vi "CRYPIC CLOSE FRAME.vi"(10 "tFrame":T2) -> ()   [LabVIEW 2013]
uses:
  <vilib>/Utility/miscctls.llb/LVRectTypeDef.ctl
  CRYMain Sub Window Global.vi
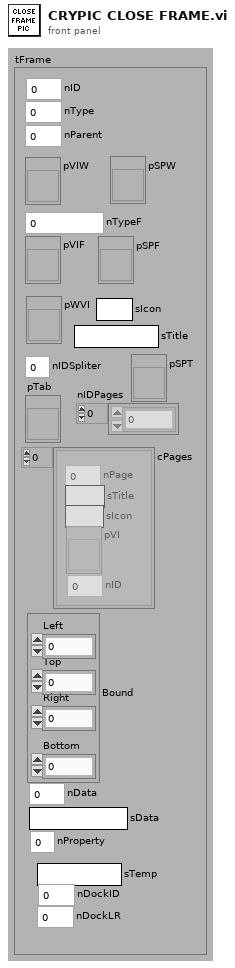
[diagram p1: front panel]
types:
  T1 = typedef "LVRectTypeDef.ctl" = cluster{"Left":i16, "Top":i16, "Right":i16, "Bottom":i16}
  T2 = cluster{"nType":i32, "nParent":i32, "pVIW":refnum<vi>, "pSPW":refnum<vi>, "nTypeF":i32, "pVIF":refnum<vi>, "pSPF":refnum<vi>, "nIDSpliter":i32, "nProperty":i32, "Bound":T1, "nID":i32, "nData":i32, "sData":string, "pWVI":refnum<vi>, "sTitle":string, "cPages":cluster{"nPage":i32, "sTitle":string, "sIcon":string, "pVI":refnum<vi>, "nID":i32}[], "pTab":refnum<vi>, "nIDPages":i32[], "pSPT":refnum<vi>, "sTemp":string, "nDockID":i32, "nDockLR":i32, "sIcon":string}
  T3 = enum32{"Invalid", "Standard", "Closed", "Hidden", "Minimized", "Maximized"}
  T4 = cluster{"nID":i32[], "Frame":cluster{"nType":i32, "nParent":i32, "pVIW":refnum<vi>, "pSPW":refnum<vi>, "nTypeF":i32, "pVIF":refnum<vi>, "pSPF":refnum<vi>, "nIDSpliter":i32, "nProperty":i32, "Bound":T1, "nID":i32, "nData":i32, "sData":string, "pWVI":refnum<vi>, "sTitle":string, "cPages":cluster{"nPage":i32, "sTitle":string, "sIcon":string, "pVI":refnum<vi>, "nID":i32}[], "pTab":refnum<vi>, "nIDPages":i32[], "pSPT":refnum<vi>, "sTemp":string, "nDockID":i32, "nDockLR":i32, "sIcon":string}[]}
  T5 = cluster{"nType":i32, "nParent":i32, "pVIW":refnum<vi>, "pSPW":refnum<vi>, "nTypeF":i32, "pVIF":refnum<vi>, "pSPF":refnum<vi>, "nIDSpliter":i32, "nProperty":i32, "Bound":T1, "nID":i32, "nData":i32, "sData":string, "pWVI":refnum<vi>, "sTitle":string, "cPages":cluster{"nPage":i32, "sTitle":string, "sIcon":string, "pVI":refnum<vi>, "nID":i32}[], "pTab":refnum<vi>, "nIDPages":i32[], "pSPT":refnum<vi>, "sTemp":string, "nDockID":i32, "nDockLR":i32, "sIcon":string}[]
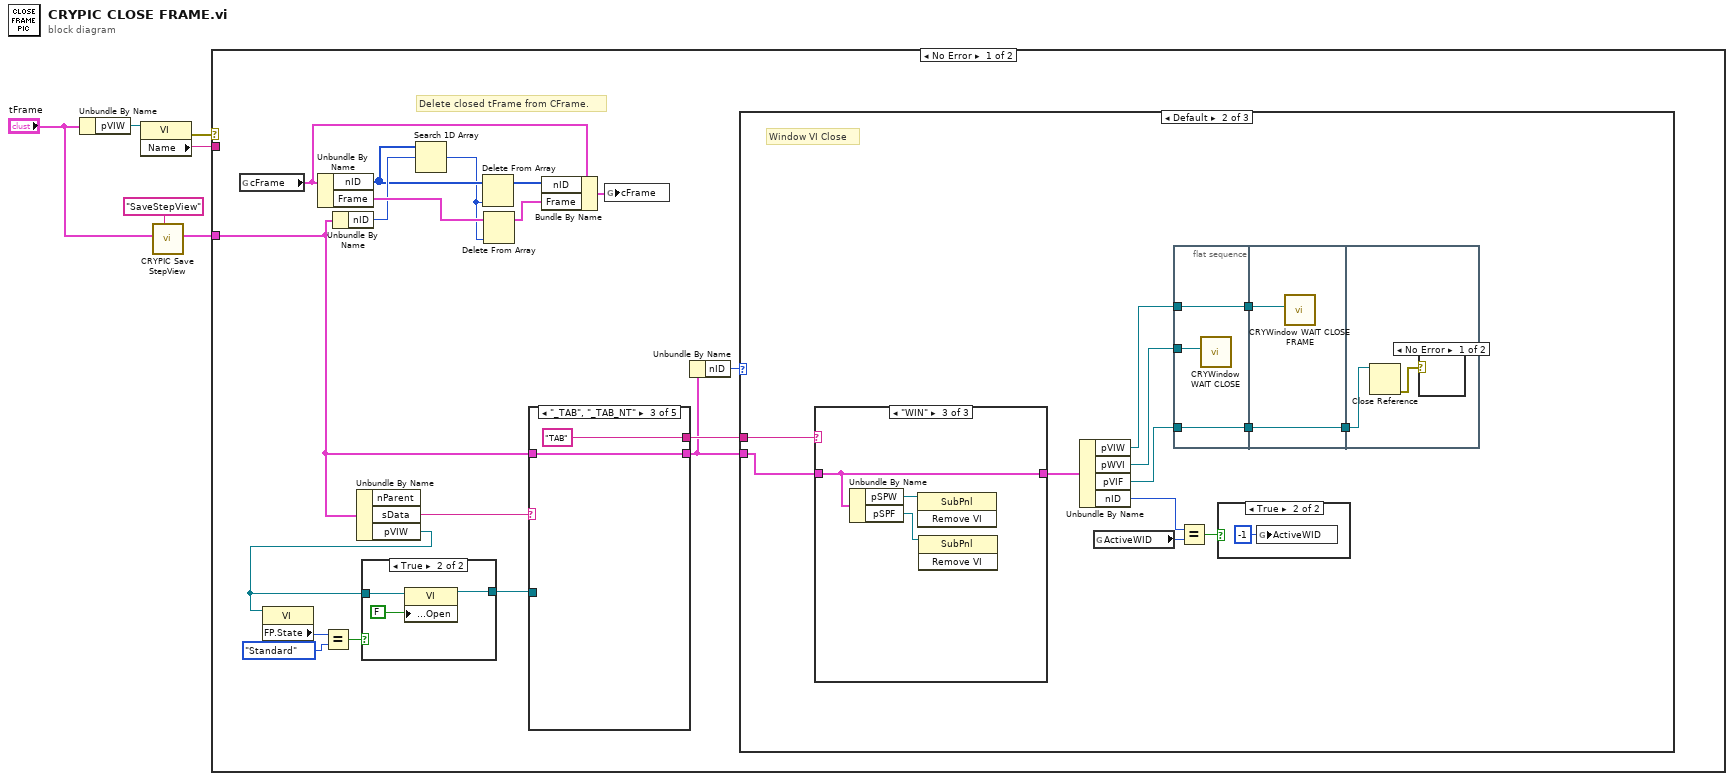
[diagram p0: block diagram]
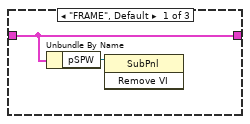
[diagram p4: hidden frame]
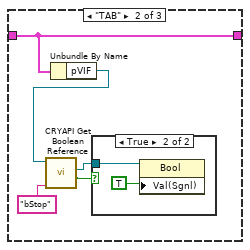
[diagram p5: hidden frame]
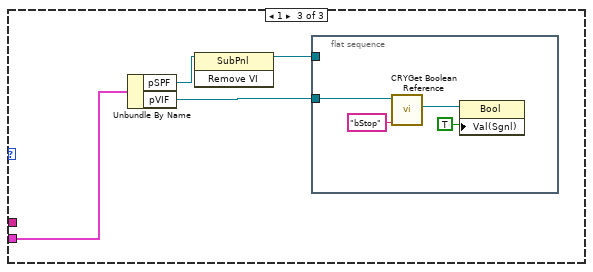
[diagram p8: hidden frame]
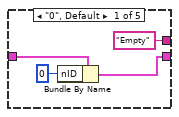
[diagram p10: hidden frame]
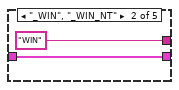
[diagram p11: hidden frame]
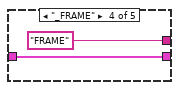
[diagram p12: hidden frame]
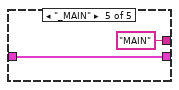
[diagram p13: hidden frame]
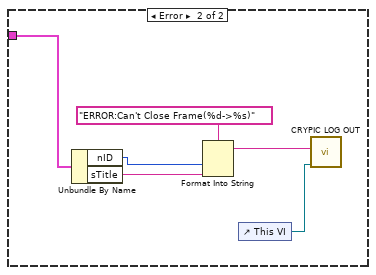
[diagram p14: hidden frame]
diagram:
  n1 = Unbundle By Name("tFrame") -> ("pVIW"=w6:refnum<vi>)
  n2 = property class="VI"(reference=w6) -> (error out=w5:errorcluster, "Name"=w4:string)  [unwired: 1 in, 1 out]
  n3 = call "CRYPIC Save StepView.vi"("sAction"="SaveStepView", "tFrame"="tFrame") -> ("tFrame_Out"=w2:T2)  [unwired: 9 in]
  n4 = case shown="No Error" w5 {
    tunnel: w4 -> [_ _]
    tunnel: w2 -> [w7 w81]
    frame No Error {
      # "Delete closed tFrame from CFrame."
      n5 = global read "CRYMain Sub Window Global.vi" "cFrame"() -> (w23:T4)
      n6 = Unbundle By Name(w23) -> ("nID"=w18:i32[], "Frame"=w24:T5)
      n7 = Unbundle By Name(w7) -> ("nID"=w19:i32)
      n8 = Unbundle By Name(w7) -> ("sData"=w11:string, "pVIW"=w12:refnum<vi>)  [unwired: 1 out]
      n9 = property class="VI"(reference=w12) -> ("FP.State"=w14:T3)  [unwired: 1 in, 2 out]
      n10 = Equal?(x=w14, y=T3."Standard" ("Front Panel Window:State")) -> (x = y?=w13:bool)
      n11 = case shown="True" w13 {
        tunnel: [w65 w67] -> w16
        tunnel: w12 -> [w65 w66]
        frame False {
        }
        frame True {
          n12 = property class="VI"(reference=w66, "Front Panel.Open"=FALSE ("Front Panel Window:Open")) -> (reference out=w67:refnum<vi>)  [unwired: 1 in, 1 out]
        }
      }
      n13 = Search 1D Array(1D array=w18, element=w19) -> (index of element=w17:i32)  [unwired: 1 out]
      n14 = Delete From Array(array=w18, index=w17) -> (array with subset deleted=w22:i32[])  [unwired: 1 in, 1 out]
      n15 = Delete From Array(array=w24, index=w17) -> (array with subset deleted=w21:T5)  [unwired: 1 in, 1 out]
      n16 = case shown="\"_TAB\", \"_TAB_NT\"" w11 {
        tunnel: w7 -> [w72 w74 w75 w77 w79]
        tunnel: [w70 w74 w75 w77 w79] -> w9
        tunnel: w16 -> [_ _ _ _ _]
        tunnel: ["Empty" ("sAction") "WIN" ("sAction") "TAB" ("sAction") "FRAME" ("sAction") "MAIN" ("sAction")] -> w10
        frame "0", Default {
          n17 = Bundle By Name(cluster=w72, "nID"=0) -> (w70:T2)
        }
        frame "_WIN", "_WIN_NT" {
        }
        frame "_TAB", "_TAB_NT" {
        }
        frame "_FRAME" {
        }
        frame "_MAIN" {
        }
      }
      n18 = Bundle By Name(cluster=w23, "nID"=w22, "Frame"=w21) -> (w20:T4)
      n19 = global write "CRYMain Sub Window Global.vi" "cFrame"(w20) -> ()
      n20 = Unbundle By Name(w9) -> ("nID"=w8:i32)
      n21 = case shown="Default" w8 {
        tunnel: w9 -> [_ w25 w60]
        tunnel: w10 -> [_ w33 _]
        frame 0 {
        }
        frame Default {
          # "Window VI Close"
          n22 = case shown="\"WIN\"" w33 {
            tunnel: w25 -> [w45 w50 w55]
            tunnel: [w45 w50 w55] -> w26
            frame "FRAME", Default {
              n23 = Unbundle By Name(w45) -> ("pSPW"=w44:refnum<vi>)
              n24 = invoke class="SubPnl" method="Remove VI"(reference=w44) -> ()  [unwired: 2 in, 3 out]
            }
            frame "TAB" {
              n25 = Unbundle By Name(w50) -> ("pVIF"=w46:refnum<vi>)
              n26 = call "CRYAPI Get Boolean Reference.vi"("Label Name"="bStop", "VI Refnum"=w46) -> ("Boolean"=w47:bool, "Boolean Ref"=w49:refnum<vi>)  [unwired: 8 out]
              n27 = case shown="True" w47 {
                tunnel: w49 -> [_ w52]
                frame False {
                }
                frame True {
                  n28 = property class="Bool"(reference=w52, "Val(Sgnl)"=TRUE) -> ()  [unwired: 1 in, 2 out]
                }
              }
            }
            frame "WIN" {
              n29 = Unbundle By Name(w55) -> ("pSPW"=w54:refnum<vi>, "pSPF"=w53:refnum<vi>)
              n30 = invoke class="SubPnl" method="Remove VI"(reference=w54) -> ()  [unwired: 2 in, 3 out]
              n31 = invoke class="SubPnl" method="Remove VI"(reference=w53) -> ()  [unwired: 2 in, 3 out]
            }
          }
          n32 = Unbundle By Name(w26) -> ("pVIW"=w31:refnum<vi>, "pWVI"=w32:refnum<vi>, "pVIF"=w29:refnum<vi>, "nID"=w36:i32)
          n33 = global read "CRYMain Sub Window Global.vi" "ActiveWID"() -> (w35:i32)
          n34 = flat-sequence {
            tunnel: w32 -> [w39]
            tunnel: w31 -> [w37]
            tunnel: [w37] -> w30
            tunnel: w29 -> [w38]
            tunnel: [w38] -> w28
            tunnel: w30 -> [w40]
            tunnel: w28 -> [w41]
            tunnel: [w41] -> w27
            tunnel: w27 -> [w42]
            frame #0 {
              n35 = call "CRYWindow WAIT CLOSE.vi"("vi reference"=w39) -> ()  [unwired: 11 in]
            }
            frame #1 {
              n36 = call "CRYWindow WAIT CLOSE FRAME.vi"("vi reference"=w40) -> ()  [unwired: 11 in]
            }
            frame #2 {
              n37 = Close Reference(reference=w42) -> (error out=w43:errorcluster)  [unwired: 1 in]
              n38 = case shown="No Error" w43 {
                frame No Error {
                }
                frame Error {
                }
              }
            }
          }
          n39 = Equal?(x=w36, y=w35) -> (x = y?=w34:bool)
          n40 = case shown="True" w34 {
            frame False {
            }
            frame True {
              n41 = global write "CRYMain Sub Window Global.vi" "ActiveWID"(-1 ("ActiveWID")) -> ()
            }
          }
        }
        frame 1 {
          n42 = Unbundle By Name(w60) -> ("pSPF"=w58:refnum<vi>, "pVIF"=w59:refnum<vi>)
          n43 = invoke class="SubPnl" method="Remove VI"(reference=w58) -> (reference out=w57:refnum<vi>)  [unwired: 2 in, 2 out]
          n44 = flat-sequence {
            tunnel: w59 -> [w61]
            tunnel: w57 -> [_]
            frame #0 {
              n45 = call "CRYGet Boolean Reference.vi"("Label Name"="bStop", "VI Refnum"=w61) -> ("Boolean Ref"=w62:refnum<vi>)  [unwired: 7 in, 2 out]
              n46 = property class="Bool"(reference=w62, "Val(Sgnl)"=TRUE) -> ()  [unwired: 1 in, 2 out]
            }
          }
        }
      }
    }
    frame Error {
      n47 = Unbundle By Name(w81) -> ("nID"=w85:i32, "sTitle"=w84:string)
      n48 = Format Into String(format string="ERROR:Can't Close Frame(%d->%s)", w85, w84) -> (resulting string=w83:string)  [unwired: 2 in, 1 out]
      n49 = control-ref of="This VI"() -> (w82:refnum<vi>)
      n50 = call "CRYPIC LOG OUT.vi"("pVIRef"=w82, "sData"=w83) -> ()  [unwired: 10 in]
    }
  }
